vi "Финал.vi"(0 "read":bool, 2 "C":bool, 3 "?":T5, 7 "Flags":T4) -> (1 "L":T1, 4 "Единицы":T2, 5 "Десятки":T2, 6 "Flags Ex":T3)   [LabVIEW 2017]
panel:
  out "_":bool
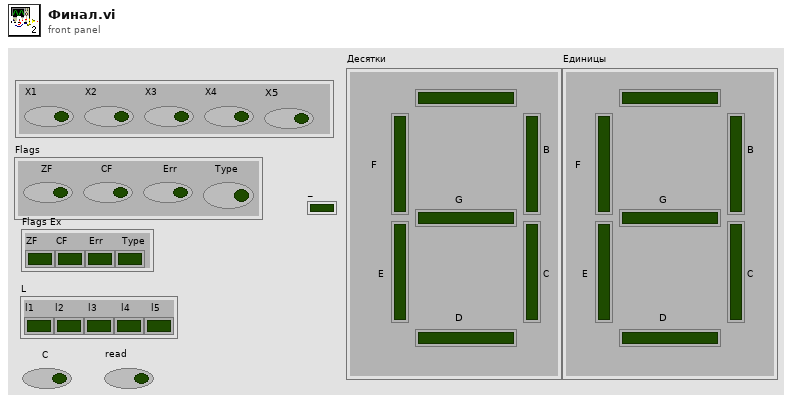
[diagram p1: front panel]
types:
  T1 = cluster{"l1":bool, "l2 ":bool, " l3":bool, "  l4":bool, "  l5":bool}
  T2 = cluster{"A":bool, "B\n ":bool, "C ":bool, "D":bool, "E ":bool, "F":bool, "G":bool}
  T3 = cluster{"ZF":bool, "CF ":bool, " Err":bool, "  Type":bool}
  T4 = cluster{"ZF":bool, "CF":bool, " Err":bool, "Type":bool}
  T5 = cluster{"X1":bool, "X2":bool, "X3":bool, "X4":bool, "X5":bool}
  T6 = cluster{"Q4":bool, "Q3":bool, "Q2":bool, "Q1":bool, "Q0":bool}
  T7 = cluster{"b 4":bool, "b 3":bool, "b 2":bool, "b 1":bool, "b 0":bool}
  T8 = cluster{"b 3":bool, "b 2":bool, "b 1":bool, "b 0":bool}
  T9 = cluster{"Q3":bool, "Q2":bool, "Q1":bool, "Q0":bool}
  T10 = cluster{"Boolean 5":bool, "Boolean 6":bool, "Boolean 7":bool, "Boolean 8":bool}
  T11 = cluster{"Boolean":bool, "Boolean 2":bool, "Boolean 3":bool, "Boolean 4":bool}
  T12 = cluster{"1":bool, "2\n ":bool, "3 ":bool, "4":bool, "5 ":bool, "6":bool, "7":bool}
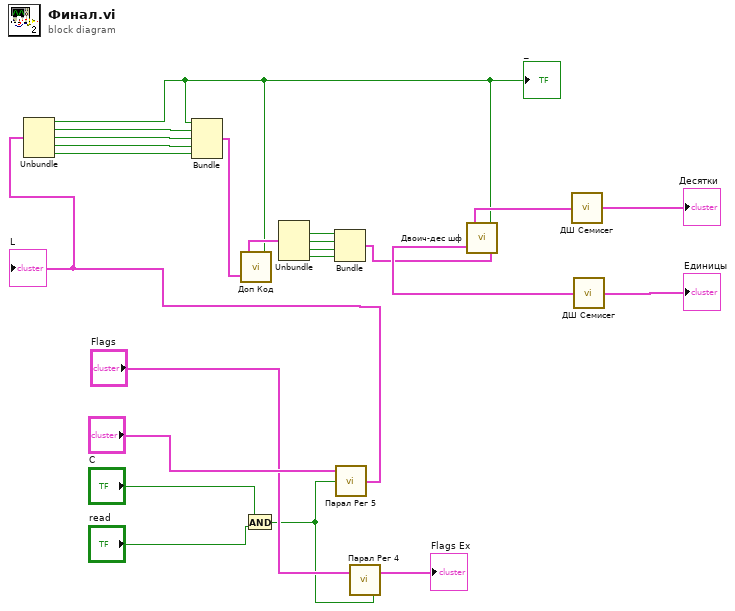
[diagram p0: block diagram]
diagram:
  n1 = And(x="C", y="read") -> (x .and. y?=w11:bool)
  n2 = call "Парал Рег 5.vi"("C"=w11, "D"="?") -> ("Q"=w3:T6)  [unwired: 1 in]
  "L" <- w3
  n3 = Unbundle(w3) -> ("Q4"=w1:bool, "Q3"=w21:bool, "Q2"=w20:bool, "Q1"=w19:bool, "Q0"=w18:bool)
  "_" <- w1
  n4 = Bundle("Q4"=w1, "Q3"=w21, "Q2"=w20, "Q1"=w19, "Q0"=w18) -> (w17:T6)  [unwired: 1 in]
  n5 = call "Доп Код.vi"("C7"=w1, "B"=w17) -> ("b"=w2:T7)
  n6 = Unbundle(w2) -> ("b 3"=w4:bool, "b 2"=w5:bool, "b 1"=w6:bool, "b 0"=w7:bool)  [unwired: 1 out]
  n7 = Bundle("b 3"=w4, "b 2"=w5, "b 1"=w6, "b 0"=w7) -> (w8:T8)  [unwired: 1 in]
  n8 = call "Парал Рег 4.vi"("C"=w11, "D"="Flags") -> ("Q"=→"Flags Ex":T9)  [unwired: 1 in]
  n9 = call "Двоич-дес шф.vi"("Registr"=w8, "Sign"=w1) -> ("Segmen 2"=w9:T10, "Segmen 1"=w10:T11)
  n10 = call "ДШ Семисег.vi"("Cluster"=w10) -> ("Cluster 2"=→"Десятки":T12)
  n11 = call "ДШ Семисег.vi"("Cluster"=w9) -> ("Cluster 2"=→"Единицы":T12)
